vi "which buttons.vi"(2 "boolean array":bool[](array[boolean]), 3 "true/false":bool) -> (0 "indexes of matching booleans":i32[](array[numeric]))   [LabVIEW 2022 SP3]
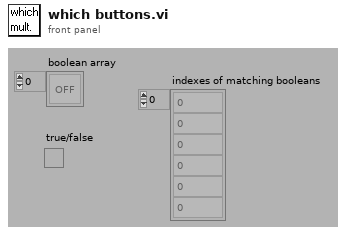
[diagram p1: front panel]
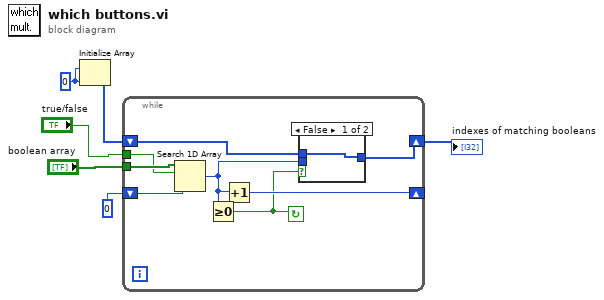
[diagram p0: block diagram]
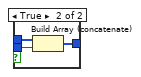
[diagram p2: hidden frame]
diagram:
  w5 = 0
  n1 = Initialize Array(w5, w5) -> (w3:i32[])
  n2 = while {
    shift-left: 0 -> [w12]
    shift-right: [w11] -> _
    tunnel: "true/false" -> [w13]
    tunnel: "boolean array" -> [w14]
    shift-left: w3 -> [w10]
    shift-right: [w8] -> w6
    stop <- w7 continue-if-true
    n3 = Search 1D Array(1D array=w14, element=w13, start index (0)=w12) -> (index of element=w9:i32)
    n4 = Greater Or Equal To 0?(x=w9) -> (x >= 0?=w7:bool)
    n5 = Increment(x=w9) -> (x+1=w11:i32)
    n6 = case shown="False" w7 {
      tunnel: w10 -> [w15 w18]
      tunnel: w9 -> [_ w17]
      tunnel: [w15 w16] -> w8
      frame False {
      }
      frame True {
        n7 = Build Array (concatenate)(w18, w17) -> (w16:i32[])
      }
    }
  }
  "indexes of matching booleans" <- w6
